vi "SplineHelp_GetQuinticCtrlVector.vi"(9 "Input POSE":T2={"TRANSLATION"={"X"=0.0, "Y"=0.0}, "ROTATION"={"VALUE"=0.0, "COS"=1.0, "SIN"=0.0}} {"ROTATION"."SIN" format="%13.4f"; "ROTATION"."COS" format="%13.4f"; "ROTATION"."VALUE" format="%13.4f"; "TRANSLATION"."Y" format="%14.3f"; "TRANSLATION"."X" format="%14.3f"}, 11 "Scalar":dbl) -> (3 "resultSpline_Ctrl_Vector":T1)   [LabVIEW 2019, in "Trajectory_Library.lvlib"]
uses:
  Trajectory_Library.lvlib
  TypeDef/SPLINE_CTRL_VECTOR.ctl
  TypeDef/TRANSLATION2D.ctl
  TypeDef/ROTATION2D.ctl
  TypeDef/POSE2D.ctl
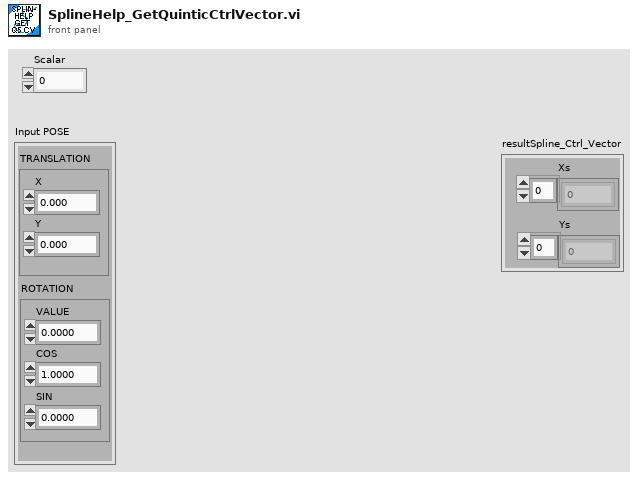
[diagram p1: front panel]
types:
  T1 = typedef "Trajectory_Library.lvlib/SPLINE_CTRL_VECTOR.ctl" = cluster{"Xs":dbl[], "Ys":dbl[]}
  T2 = typedef "Trajectory_Library.lvlib/POSE2D.ctl" = cluster{"TRANSLATION":T3, "ROTATION":T4}
  T3 = typedef "Trajectory_Library.lvlib/TRANSLATION2D.ctl" = cluster{"X":dbl, "Y":dbl}
  T4 = typedef "Trajectory_Library.lvlib/ROTATION2D.ctl" = cluster{"VALUE":dbl, "COS":dbl, "SIN":dbl}
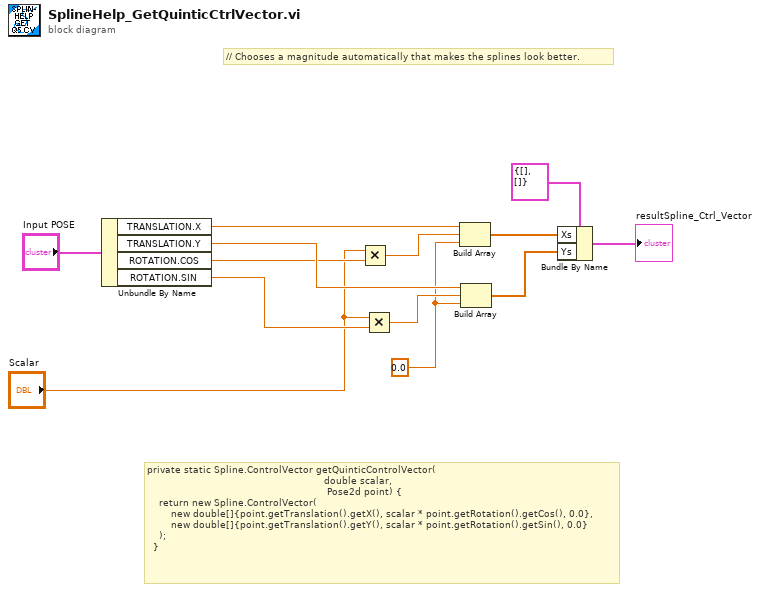
[diagram p0: block diagram]
diagram:
  w1 = 0.0
  # "private static Spline.ControlVector getQuinticControlVector(\n                                                           double scalar, \n                                                            Pose2d point) {\n    return new Spline.ControlVector(\n        new double[]{point.getTranslation().getX(), scalar * point.getRotation().getCos(), 0.0},\n        new double[]{point.getTranslation().getY(), scalar * point.getRotation().getSin(), 0.0}\n    );\n  }"
  # "// Chooses a magnitude automatically that makes the splines look better."
  n1 = Unbundle By Name("Input POSE") -> ("TRANSLATION.X"=w8:dbl, "TRANSLATION.Y"=w7:dbl, "ROTATION.COS"=w6:dbl, "ROTATION.SIN"=w5:dbl)
  n2 = Multiply(x="Scalar", y=w6) -> (x*y=w3:dbl)
  n3 = Multiply(x="Scalar", y=w5) -> (x*y=w2:dbl)
  n4 = Build Array(w8, w3, w1) -> (w11:dbl[])
  n5 = Build Array(w7, w2, w1) -> (w10:dbl[])
  n6 = Bundle By Name(cluster=T1 {"Xs"=[], "Ys"=[]} ("SPLINE_CTRL_VECTOR"), "Xs"=w11, "Ys"=w10) -> (→"resultSpline_Ctrl_Vector":T1)
